vi "SingleTempUpdater.vi"(3 "Well Coordinates":T2[](array[typedef])=[{"X"=62.0, "Y"=66.0}, {"X"=77.521736, "Y"=65.73913}, {"X"=93.04348, "Y"=65.478264}, {"X"=108.565216, "Y"=65.21739}, {"X"=124.08696, "Y"=64.95652}, {"X"=139.6087, "Y"=64.695656}, {"X"=155.13043, "Y"=64.434784}, {"X"=170.65218, "Y"=64.17391}, {"X"=186.17392, "Y"=63.913044}, {"X"=201.69565, "Y"=63.652176}, {"X"=217.21739, "Y"=63.391304}, {"X"=232.73914, "Y"=63.130436}, {"X"=248.26086, "Y"=62.869564}, {"X"=263.7826, "Y"=62.608696}, {"X"=279.30435, "Y"=62.347824}, {"X"=294.82608, "Y"=62.086956}, {"X"=310.34784, "Y"=61.826088}, {"X"=325.86957, "Y"=61.565216}, {"X"=341.3913, "Y"=61.304348}, {"X"=356.91306, "Y"=61.04348}, {"X"=372.43478, "Y"=60.782608}, {"X"=387.9565, "Y"=60.52174}, {"X"=403.47827, "Y"=60.260868}, {"X"=419.0, "Y"=60.0}, {"X"=62.333332, "Y"=81.53333}, {"X"=77.85507, "Y"=81.27246}, {"X"=93.37681, "Y"=81.0116}, {"X"=108.89855, "Y"=80.750725}, {"X"=124.42029, "Y"=80.48985}, {"X"=139.94203, "Y"=80.22899}, {"X"=155.46376, "Y"=79.96812}, {"X"=170.9855, "Y"=79.707245}, {"X"=186.50725, "Y"=79.44638}, {"X"=202.02898, "Y"=79.18551}, {"X"=217.55072, "Y"=78.92464}, {"X"=233.07246, "Y"=78.66377}, {"X"=248.5942, "Y"=78.4029}, {"X"=264.11594, "Y"=78.14203}, {"X"=279.6377, "Y"=77.88116}, {"X"=295.15942, "Y"=77.62029}, {"X"=310.68115, "Y"=77.35942}, {"X"=326.2029, "Y"=77.09855}, {"X"=341.72464, "Y"=76.837685}, {"X"=357.2464, "Y"=76.57681}, {"X"=372.76813, "Y"=76.31594}, {"X"=388.28986, "Y"=76.05507}, {"X"=403.8116, "Y"=75.794205}, {"X"=419.33334, "Y"=75.53333}, {"X"=62.666668, "Y"=97.066666}, {"X"=78.18841, "Y"=96.8058}, {"X"=93.710144, "Y"=96.54493}, {"X"=109.23188, "Y"=96.28406}, {"X"=124.753624, "Y"=96.02319}, {"X"=140.27536, "Y"=95.76232}, {"X"=155.7971, "Y"=95.50145}, {"X"=171.31885, "Y"=95.240585}, {"X"=186.84058, "Y"=94.97971}, {"X"=202.36232, "Y"=94.71884}, {"X"=217.88406, "Y"=94.45797}, {"X"=233.4058, "Y"=94.1971}, {"X"=248.92754, "Y"=93.93623}, {"X"=264.44928, "Y"=93.67536}, {"X"=279.971, "Y"=93.41449}, {"X"=295.49274, "Y"=93.153625}, {"X"=311.0145, "Y"=92.89275}, {"X"=326.53622, "Y"=92.63188}, {"X"=342.05795, "Y"=92.37102}, {"X"=357.5797, "Y"=92.110146}, {"X"=373.10144, "Y"=91.84927}, {"X"=388.62317, "Y"=91.58841}, {"X"=404.14493, "Y"=91.32754}, {"X"=419.66666, "Y"=91.066666}, {"X"=63.0, "Y"=112.600006}, {"X"=78.521736, "Y"=112.339134}, {"X"=94.04348, "Y"=112.07826}, {"X"=109.565216, "Y"=111.8174}, {"X"=125.08696, "Y"=111.55652}, {"X"=140.6087, "Y"=111.295654}, {"X"=156.13043, "Y"=111.03479}, {"X"=171.65218, "Y"=110.77391}, {"X"=187.17392, "Y"=110.51305}, {"X"=202.69565, "Y"=110.252174}, {"X"=218.21739, "Y"=109.9913}, {"X"=233.73914, "Y"=109.73044}, {"X"=249.26086, "Y"=109.46957}, {"X"=264.78262, "Y"=109.208694}, {"X"=280.30435, "Y"=108.94783}, {"X"=295.82608, "Y"=108.68696}, {"X"=311.34784, "Y"=108.42609}, {"X"=326.86957, "Y"=108.16522}, {"X"=342.3913, "Y"=107.90435}, {"X"=357.91306, "Y"=107.64348}, {"X"=373.43478, "Y"=107.382614}, {"X"=388.9565, "Y"=107.12174}, {"X"=404.47827, "Y"=106.86087}, {"X"=420.0, "Y"=106.600006}, {"X"=63.333332, "Y"=128.13333}, {"X"=78.85507, "Y"=127.87247}, {"X"=94.37681, "Y"=127.611595}, {"X"=109.89855, "Y"=127.35072}, {"X"=125.42029, "Y"=127.08986}, {"X"=140.94203, "Y"=126.82899}, {"X"=156.46376, "Y"=126.568115}, {"X"=171.9855, "Y"=126.30725}, {"X"=187.50725, "Y"=126.04638}, {"X"=203.02898, "Y"=125.78551}, {"X"=218.55072, "Y"=125.52464}, {"X"=234.07246, "Y"=125.26377}, {"X"=249.5942, "Y"=125.0029}, {"X"=265.11594, "Y"=124.742035}, {"X"=280.6377, "Y"=124.48116}, {"X"=296.15942, "Y"=124.22029}, {"X"=311.68115, "Y"=123.95943}, {"X"=327.2029, "Y"=123.69855}, {"X"=342.72464, "Y"=123.43768}, {"X"=358.2464, "Y"=123.17682}, {"X"=373.76813, "Y"=122.91594}, {"X"=389.28986, "Y"=122.655075}, {"X"=404.8116, "Y"=122.3942}, {"X"=420.33334, "Y"=122.13333}, {"X"=63.666668, "Y"=143.66667}, {"X"=79.18841, "Y"=143.40579}, {"X"=94.710144, "Y"=143.14493}, {"X"=110.23188, "Y"=142.88406}, {"X"=125.753624, "Y"=142.6232}, {"X"=141.27536, "Y"=142.36234}, {"X"=156.7971, "Y"=142.10146}, {"X"=172.31885, "Y"=141.84058}, {"X"=187.84058, "Y"=141.57971}, {"X"=203.36232, "Y"=141.31885}, {"X"=218.88406, "Y"=141.05798}, {"X"=234.4058, "Y"=140.7971}, {"X"=249.92754, "Y"=140.53624}, {"X"=265.44928, "Y"=140.27536}, {"X"=280.971, "Y"=140.0145}, {"X"=296.49274, "Y"=139.75363}, {"X"=312.0145, "Y"=139.49277}, {"X"=327.53622, "Y"=139.23189}, {"X"=343.05795, "Y"=138.97102}, {"X"=358.5797, "Y"=138.71014}, {"X"=374.10144, "Y"=138.44928}, {"X"=389.62317, "Y"=138.18842}, {"X"=405.14493, "Y"=137.92755}, {"X"=420.66666, "Y"=137.66667}, {"X"=64.0, "Y"=159.20001}, {"X"=79.521736, "Y"=158.93913}, {"X"=95.04348, "Y"=158.67827}, {"X"=110.565216, "Y"=158.41739}, {"X"=126.08696, "Y"=158.15652}, {"X"=141.6087, "Y"=157.89566}, {"X"=157.13043, "Y"=157.6348}, {"X"=172.65218, "Y"=157.37392}, {"X"=188.17392, "Y"=157.11304}, {"X"=203.69565, "Y"=156.85217}, {"X"=219.21739, "Y"=156.59131}, {"X"=234.73914, "Y"=156.33044}, {"X"=250.26086, "Y"=156.06958}, {"X"=265.78262, "Y"=155.8087}, {"X"=281.30435, "Y"=155.54782}, {"X"=296.82608, "Y"=155.28696}, {"X"=312.34784, "Y"=155.0261}, {"X"=327.86957, "Y"=154.76523}, {"X"=343.3913, "Y"=154.50435}, {"X"=358.91306, "Y"=154.24348}, {"X"=374.43478, "Y"=153.9826}, {"X"=389.9565, "Y"=153.72174}, {"X"=405.47827, "Y"=153.46088}, {"X"=421.0, "Y"=153.20001}, {"X"=64.333336, "Y"=174.73334}, {"X"=79.85507, "Y"=174.47247}, {"X"=95.37681, "Y"=174.21161}, {"X"=110.89855, "Y"=173.95073}, {"X"=126.42029, "Y"=173.68985}, {"X"=141.94203, "Y"=173.42899}, {"X"=157.46376, "Y"=173.16812}, {"X"=172.9855, "Y"=172.90726}, {"X"=188.50725, "Y"=172.64638}, {"X"=204.02898, "Y"=172.38551}, {"X"=219.55072, "Y"=172.12463}, {"X"=235.07246, "Y"=171.86377}, {"X"=250.5942, "Y"=171.6029}, {"X"=266.11594, "Y"=171.34204}, {"X"=281.6377, "Y"=171.08116}, {"X"=297.15942, "Y"=170.8203}, {"X"=312.68115, "Y"=170.55942}, {"X"=328.2029, "Y"=170.29855}, {"X"=343.72464, "Y"=170.03769}, {"X"=359.2464, "Y"=169.77682}, {"X"=374.76813, "Y"=169.51595}, {"X"=390.28986, "Y"=169.25507}, {"X"=405.8116, "Y"=168.9942}, {"X"=421.33334, "Y"=168.73334}, {"X"=64.666664, "Y"=190.26666}, {"X"=80.18841, "Y"=190.0058}, {"X"=95.710144, "Y"=189.74493}, {"X"=111.23188, "Y"=189.48407}, {"X"=126.753624, "Y"=189.22319}, {"X"=142.27536, "Y"=188.96233}, {"X"=157.7971, "Y"=188.70145}, {"X"=173.31885, "Y"=188.44058}, {"X"=188.84058, "Y"=188.17972}, {"X"=204.36232, "Y"=187.91885}, {"X"=219.88406, "Y"=187.65797}, {"X"=235.4058, "Y"=187.3971}, {"X"=250.92754, "Y"=187.13623}, {"X"=266.44928, "Y"=186.87537}, {"X"=281.971, "Y"=186.6145}, {"X"=297.49274, "Y"=186.35364}, {"X"=313.0145, "Y"=186.09276}, {"X"=328.53622, "Y"=185.83188}, {"X"=344.05795, "Y"=185.57101}, {"X"=359.5797, "Y"=185.31015}, {"X"=375.10144, "Y"=185.04929}, {"X"=390.62317, "Y"=184.7884}, {"X"=406.14493, "Y"=184.52754}, {"X"=421.66666, "Y"=184.26666}, {"X"=65.0, "Y"=205.8}, {"X"=80.521736, "Y"=205.53914}, {"X"=96.04348, "Y"=205.27826}, {"X"=111.565216, "Y"=205.0174}, {"X"=127.08696, "Y"=204.75653}, {"X"=142.6087, "Y"=204.49565}, {"X"=158.13043, "Y"=204.23479}, {"X"=173.65218, "Y"=203.97392}, {"X"=189.17392, "Y"=203.71304}, {"X"=204.69565, "Y"=203.45218}, {"X"=220.21739, "Y"=203.19131}, {"X"=235.73914, "Y"=202.93044}, {"X"=251.26086, "Y"=202.66957}, {"X"=266.78262, "Y"=202.40869}, {"X"=282.30435, "Y"=202.14783}, {"X"=297.82608, "Y"=201.88696}, {"X"=313.34784, "Y"=201.62608}, {"X"=328.86957, "Y"=201.36522}, {"X"=344.3913, "Y"=201.10435}, {"X"=359.91306, "Y"=200.84348}, {"X"=375.43478, "Y"=200.58261}, {"X"=390.9565, "Y"=200.32175}, {"X"=406.47827, "Y"=200.06087}, {"X"=422.0, "Y"=199.8}, {"X"=65.333336, "Y"=221.33334}, {"X"=80.85507, "Y"=221.07248}, {"X"=96.37681, "Y"=220.8116}, {"X"=111.89855, "Y"=220.55074}, {"X"=127.42029, "Y"=220.28987}, {"X"=142.94203, "Y"=220.02899}, {"X"=158.46376, "Y"=219.76813}, {"X"=173.9855, "Y"=219.50726}, {"X"=189.50725, "Y"=219.24638}, {"X"=205.02898, "Y"=218.98552}, {"X"=220.55072, "Y"=218.72466}, {"X"=236.07246, "Y"=218.46378}, {"X"=251.5942, "Y"=218.20291}, {"X"=267.11594, "Y"=217.94203}, {"X"=282.6377, "Y"=217.68117}, {"X"=298.15942, "Y"=217.4203}, {"X"=313.68115, "Y"=217.15942}, {"X"=329.2029, "Y"=216.89856}, {"X"=344.72464, "Y"=216.6377}, {"X"=360.2464, "Y"=216.37682}, {"X"=375.76813, "Y"=216.11595}, {"X"=391.28986, "Y"=215.85509}, {"X"=406.8116, "Y"=215.59421}, {"X"=422.33334, "Y"=215.33334}, {"X"=65.666664, "Y"=236.86667}, {"X"=81.18841, "Y"=236.6058}, {"X"=96.710144, "Y"=236.34492}, {"X"=112.23188, "Y"=236.08406}, {"X"=127.753624, "Y"=235.8232}, {"X"=143.27536, "Y"=235.56232}, {"X"=158.7971, "Y"=235.30145}, {"X"=174.31885, "Y"=235.04059}, {"X"=189.84058, "Y"=234.77971}, {"X"=205.36232, "Y"=234.51884}, {"X"=220.88406, "Y"=234.25798}, {"X"=236.4058, "Y"=233.9971}, {"X"=251.92754, "Y"=233.73624}, {"X"=267.44928, "Y"=233.47536}, {"X"=282.971, "Y"=233.2145}, {"X"=298.49274, "Y"=232.95363}, {"X"=314.0145, "Y"=232.69275}, {"X"=329.53622, "Y"=232.43188}, {"X"=345.05795, "Y"=232.17102}, {"X"=360.5797, "Y"=231.91014}, {"X"=376.10144, "Y"=231.64928}, {"X"=391.62317, "Y"=231.38841}, {"X"=407.14493, "Y"=231.12753}, {"X"=422.66666, "Y"=230.86667}, {"X"=66.0, "Y"=252.40001}, {"X"=81.521736, "Y"=252.13914}, {"X"=97.04348, "Y"=251.87827}, {"X"=112.565216, "Y"=251.6174}, {"X"=128.08696, "Y"=251.35654}, {"X"=143.6087, "Y"=251.09566}, {"X"=159.13043, "Y"=250.8348}, {"X"=174.65218, "Y"=250.57393}, {"X"=190.17392, "Y"=250.31305}, {"X"=205.69565, "Y"=250.05219}, {"X"=221.21739, "Y"=249.79132}, {"X"=236.73914, "Y"=249.53044}, {"X"=252.26086, "Y"=249.26958}, {"X"=267.78262, "Y"=249.0087}, {"X"=283.30435, "Y"=248.74783}, {"X"=298.82608, "Y"=248.48697}, {"X"=314.34784, "Y"=248.22609}, {"X"=329.86957, "Y"=247.96523}, {"X"=345.3913, "Y"=247.70436}, {"X"=360.91306, "Y"=247.44348}, {"X"=376.43478, "Y"=247.18262}, {"X"=391.9565, "Y"=246.92175}, {"X"=407.47827, "Y"=246.66087}, {"X"=423.0, "Y"=246.40001}, {"X"=66.333336, "Y"=267.93335}, {"X"=81.85507, "Y"=267.6725}, {"X"=97.37681, "Y"=267.4116}, {"X"=112.89855, "Y"=267.15073}, {"X"=128.42029, "Y"=266.88986}, {"X"=143.94203, "Y"=266.62897}, {"X"=159.46376, "Y"=266.3681}, {"X"=174.9855, "Y"=266.10724}, {"X"=190.50725, "Y"=265.84637}, {"X"=206.02898, "Y"=265.5855}, {"X"=221.55072, "Y"=265.32465}, {"X"=237.07246, "Y"=265.06378}, {"X"=252.5942, "Y"=264.80292}, {"X"=268.11594, "Y"=264.54202}, {"X"=283.6377, "Y"=264.28116}, {"X"=299.15942, "Y"=264.0203}, {"X"=314.68115, "Y"=263.7594}, {"X"=330.2029, "Y"=263.49854}, {"X"=345.72464, "Y"=263.23767}, {"X"=361.2464, "Y"=262.9768}, {"X"=376.76813, "Y"=262.71594}, {"X"=392.28986, "Y"=262.45508}, {"X"=407.8116, "Y"=262.1942}, {"X"=423.33334, "Y"=261.93335}, {"X"=66.666664, "Y"=283.46667}, {"X"=82.18841, "Y"=283.2058}, {"X"=97.710144, "Y"=282.94495}, {"X"=113.23188, "Y"=282.68408}, {"X"=128.75362, "Y"=282.42322}, {"X"=144.27536, "Y"=282.16232}, {"X"=159.7971, "Y"=281.90146}, {"X"=175.31885, "Y"=281.6406}, {"X"=190.84058, "Y"=281.3797}, {"X"=206.36232, "Y"=281.11884}, {"X"=221.88406, "Y"=280.85797}, {"X"=237.4058, "Y"=280.5971}, {"X"=252.92754, "Y"=280.33624}, {"X"=268.44928, "Y"=280.07538}, {"X"=283.971, "Y"=279.8145}, {"X"=299.49274, "Y"=279.55365}, {"X"=315.0145, "Y"=279.29276}, {"X"=330.53622, "Y"=279.0319}, {"X"=346.05795, "Y"=278.77103}, {"X"=361.5797, "Y"=278.51013}, {"X"=377.10144, "Y"=278.24927}, {"X"=392.62317, "Y"=277.9884}, {"X"=408.14493, "Y"=277.72754}, {"X"=423.66666, "Y"=277.46667}, {"X"=67.0, "Y"=299.0}, {"X"=82.521736, "Y"=298.73914}, {"X"=98.04348, "Y"=298.47827}, {"X"=113.565216, "Y"=298.2174}, {"X"=129.08696, "Y"=297.95654}, {"X"=144.6087, "Y"=297.69565}, {"X"=160.13043, "Y"=297.43478}, {"X"=175.65218, "Y"=297.17392}, {"X"=191.17392, "Y"=296.91302}, {"X"=206.69565, "Y"=296.65216}, {"X"=222.21739, "Y"=296.3913}, {"X"=237.73914, "Y"=296.13043}, {"X"=253.26086, "Y"=295.86957}, {"X"=268.78262, "Y"=295.6087}, {"X"=284.30435, "Y"=295.34784}, {"X"=299.82608, "Y"=295.08698}, {"X"=315.34784, "Y"=294.82608}, {"X"=330.86957, "Y"=294.56522}, {"X"=346.3913, "Y"=294.30435}, {"X"=361.91306, "Y"=294.04346}, {"X"=377.43478, "Y"=293.7826}, {"X"=392.9565, "Y"=293.52173}, {"X"=408.47827, "Y"=293.26086}, {"X"=424.0, "Y"=293.0}] {"Y" format="%.2f"; "X" format="%.2f"}, 4 "Well idx":i32, 5 "Valid Point?":bool) -> (0 "Well idx":i32, 1 "ROI Descriptor":T1 {"Contours"."Type" items=["No Selection", "Point", "Line", "Rectangle", "Oval", "Polygon", "Freehand Region", "Annulus", "Unused2", "Unused3", "Broken Line", "Freehand Line", "Rotated Rectangle"]}, 2 "State out":string)   [LabVIEW 2021]
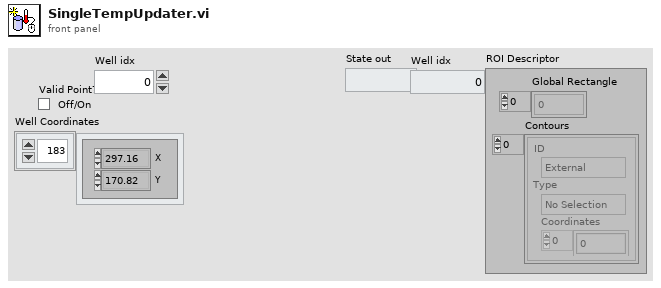
[diagram p1: front panel]
types:
  T1 = typedef "ROI Descriptor" = cluster{"Global Rectangle":i32[], "Contours":cluster{"ID":enum32{"External", "Internal"}, "Type":u32, "Coordinates":i32[]}[]}
  T2 = typedef "IMAQ Point" = cluster{"X":sgl, "Y":sgl}
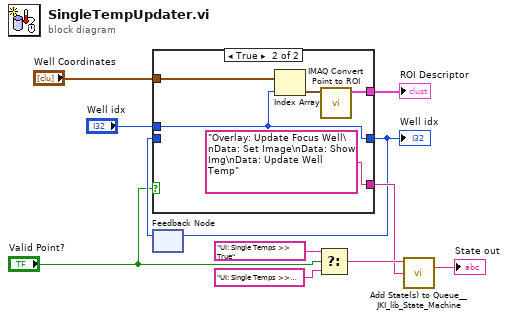
[diagram p0: block diagram]
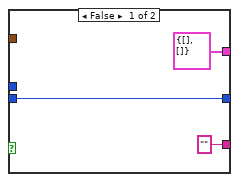
[diagram p2: hidden frame]
diagram:
  n1 = feedback #1() -> (w7:i32)  [unwired: 1 in]
  n2 = case shown="True" "Valid Point?" {
    tunnel: "Well idx" -> [_ w15]
    tunnel: [w13 w15] -> w6
    tunnel: ["" ("f") "Overlay: Update Focus Well\nData: Set Image\nData: Show Img\nData: Update Well Temp"] -> w9
    tunnel: w7 -> [w13 _]
    tunnel: "Well Coordinates" -> [_ w17]
    tunnel: [T1 {"Global Rectangle"=[], "Contours"=[]} ("ROI Descriptor") w16] -> w4
    frame False {
    }
    frame True {
      n3 = Index Array(array=w17, index=w15) -> (element=w18:T2)
      n4 = call "IMAQ Convert Point to ROI"("Point"=w18) -> ("ROI Descriptor"=w16:T1)  [unwired: 8 in, 1 out]
    }
  }
  "Well idx" <- w6
  "ROI Descriptor" <- w4
  n5 = feedback-in #1(w6) -> ()
  n6 = Select(t="UI: Single Temps >> True", s="Valid Point?", f="UI: Single Temps >> False") -> (s? t:f=w10:string)
  n7 = call <vilib>:"Add State(s) to Queue__JKI_lib_State_Machine.vi"("State(s) in Front (\"\")"=w10, "State(s) at Back (\"\")"=w9) -> ("States Out"=→"State out":string)  [unwired: 13 in]
